vi "RichToFlatnixnet_grpc_EptRxFilterArray.vi"(5 "OutputClusterType":T1, 11 "InputCluster":T3) -> (3 "OutputCluster":T1)   [LabVIEW 2024, in "grpc-xnet_client.lvlib"]
uses:
  grpc-xnet_client.lvlib
  nixnet_grpc_EptRxFilter_Flat.ctl
  nixnet_grpc_EptRxFilterArray_Flat.ctl
  nixnet_grpc_EptRxFilter.ctl
  nixnet_grpc_EptRxFilterArray.ctl
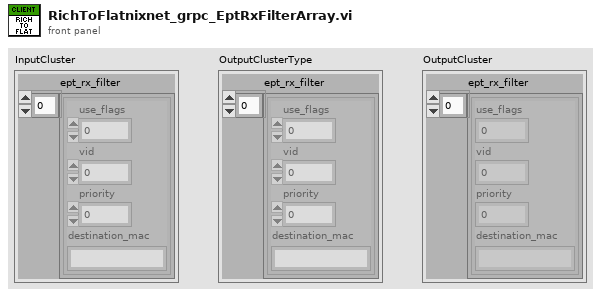
[diagram p1: front panel]
types:
  T1 = typedef "grpc-xnet_client.lvlib/nixnet_grpc_EptRxFilterArray_Flat.ctl" = cluster{"ept_rx_filter":T2[]}
  T2 = typedef "grpc-xnet_client.lvlib/nixnet_grpc_EptRxFilter_Flat.ctl" = cluster{"use_flags":u32, "vid":u32, "priority":u32, "destination_mac":string}
  T3 = typedef "grpc-xnet_client.lvlib/nixnet_grpc_EptRxFilterArray.ctl" = cluster{"ept_rx_filter":T4[]}
  T4 = typedef "grpc-xnet_client.lvlib/nixnet_grpc_EptRxFilter.ctl" = cluster{"use_flags":u32, "vid":u32, "priority":u32, "destination_mac":string}
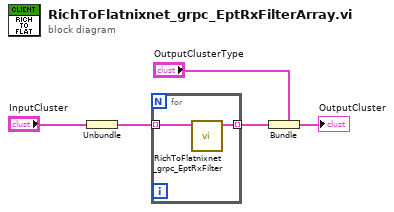
[diagram p0: block diagram]
diagram:
  n1 = Unbundle "Unbundle"("InputCluster") -> ("ept_rx_filter"=w2:T4[])
  n2 = for {
    tunnel: w2 -> [w7] mode=indexing
    tunnel: [w6] -> w1 mode=indexing
    n3 = call "RichToFlatnixnet_grpc_EptRxFilter.vi"("InputCluster"=w7) -> ("OutputCluster"=w6:T2)  [unwired: 10 in]
  }
  n4 = Bundle "Bundle"(cluster="OutputClusterType", "ept_rx_filter"=w1) -> (→"OutputCluster":T1)
